vi "example_8bit_target.vi"() -> ()   [LabVIEW 2013]
uses:
  <vilib>/Platform/TimedLoop/XDataNode/wakeup.ctl
  <vilib>/Platform/TimedLoop/XDataNode/XDNodeRunTimeDep.lvlib
  <vilib>/Platform/TimedLoop/XDataNode/nitl_modes.ctl
  <vilib>/Platform/TimedLoop/XDataNode/timing_clust.ctl
  <vilib>/Platform/TimedLoop/XDataNode/XDataNode.xnode
  <vilib>/rvi/DataTransferAndStorage/Container/XNode/niFpgaContainer.xnode
  <vilib>/rvi/Memory/Memory_Emulation/niFpgaMemoryEmulationDramWriteAndRequestDataRefIn.vi
  <vilib>/eio/EIONode/EIONode.xnode
  <vilib>/rvi/eio/common/nirviEmuTemplateMethod_errors.vi
  <vilib>/rvi/FIFO/Fifo_Resource/niFpgaFifoEmulationRefIn.vi
panel:
  in  "Load":bool
  in  "Стоп":bool
  in  "Check":bool
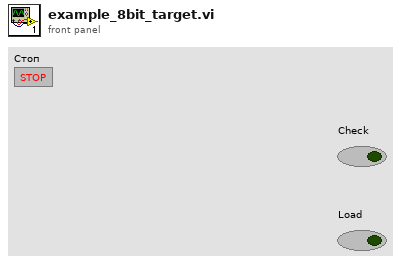
[diagram p1: front panel]
types:
  T1 = typedef "XDNodeRunTimeDep.lvlib/timing_clust.ctl" = cluster{"Expected End [f-1]":u64, "Actual End [f-1]":u64, "Finished Late? [f-1]":bool, "Expected End [i-1]":u64, "Actual End [i-1]":u64, "Finished Late? [i-1]":bool, "Expected Start [i]":u64, "Actual Start [i]":u64, "Expected Start [f]":u64, "Actual Start [f]":u64, "Source Name":string, "Structure Name":string, "Period":i64, "Deadline":i64, "Offset":i64, "Start":i64, "Priority":i32, "Timeout":i32, "Mode":T2, "Wakeup Reason":T3, "Error":errorcluster, "Source Type":string, "Secondary Source Type":string, "Global End Time":u64, "Global Start Time":u64, "Frame Duration":u64, "Iteration Duration":u64, "Assigned CPU":i32, "I/O Scan Engine Mode":u32}
  T2 = typedef "XDNodeRunTimeDep.lvlib/nitl_modes.ctl" = enum32{"No Change", "Process missed periods, maintain original phase", "Discard missed periods, maintain original phase", "Process missed periods, ignore original phase", "Discard missed periods, ignore original phase"}
  T3 = typedef "XDNodeRunTimeDep.lvlib/wakeup.ctl" = enum32{"Normal", "Aborted", "Asynchronous wakeup", "Timing source error", "Timed loop error", "Timeout"}
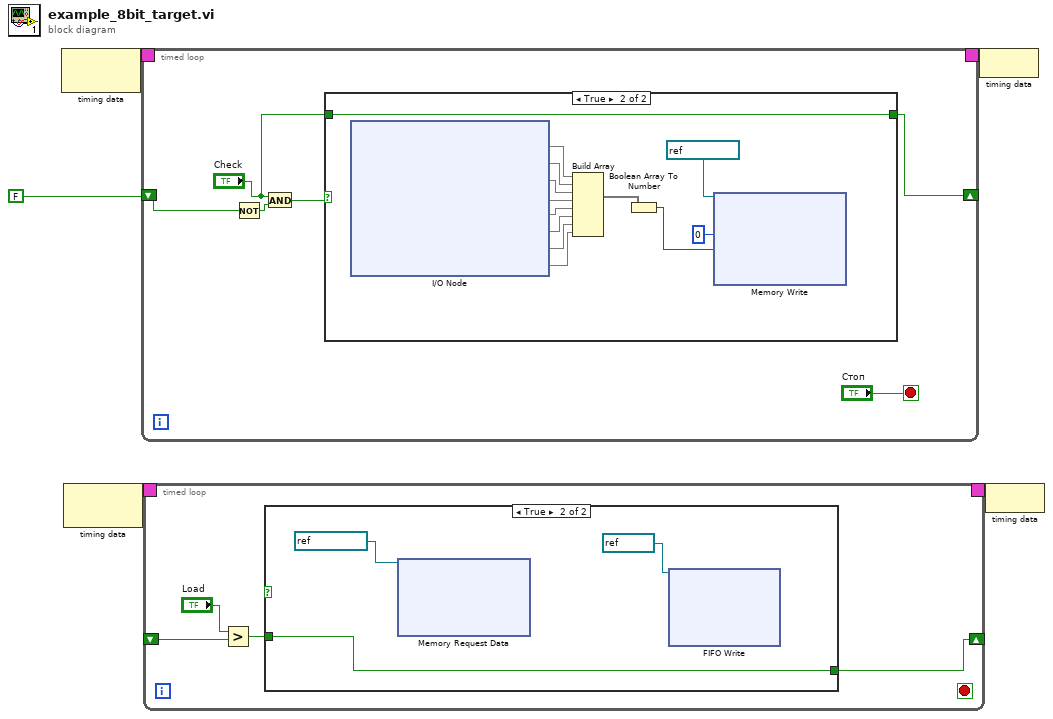
[diagram p0: block diagram]
diagram:
  n1 = node-c288() -> (w5:T1)  [unwired: 1 in]
  n2 = node-c288() -> (w3:T1)  [unwired: 1 in]
  n3 = timed-loop {
    timing: w5 -> [_]
    timing-out: [_] -> w4
    shift-right: [w7] -> _
    shift-left: FALSE -> [w8]
    stop <- "Стоп" stop-if-true
    n4 = Not(x=w8) -> (.not. x?=w9:bool)
    n5 = And(x="Check", y=w9) -> (x .and. y?=w10:bool)
    n6 = case shown="True" w10 {
      tunnel: [w12 w17] -> w7
      tunnel: "Check" -> [w12 w17]
      frame False {
      }
      frame True {
        n7 = xnode "I/O Node"() -> ("IO Module\\DDCA_DIO0_Read"=w25, "IO Module\\DDCA_DIO1_Read"=w24, "IO Module\\DDCA_DIO2_Read"=w23, "IO Module\\DDCA_DIO3_Read"=w22, "IO Module\\DDCA_DIO4_Read"=w21, "IO Module\\DDCA_DIO5_Read"=w20, "IO Module\\DDCA_DIO6_Read"=w19, "IO Module\\DDCA_DIO7_Read"=w18)  [unwired: 8 in, 8 out]
        n8 = Build Array(w25, w24, w23, w22, w21, w20, w19, w18) -> (w13:void[])
        n9 = Boolean Array To Number(Boolean array=w13) -> (number=w15:u32)
        n10 = xnode "Memory Write"("Address"=u32 0, "Data"=w15, "Memory In"=refnum<k21> "Memory") -> ()  [unwired: 1 in, 2 out]
      }
    }
  }
  n11 = timed-loop {
    timing: w3 -> [_]
    timing-out: [_] -> w2
    shift-right: [w30] -> _
    shift-left: _ -> [w28]
    stop <- _ stop-if-true
    n12 = Greater?(x="Load", y=w28) -> (0:w29:bool)
    n13 = case shown="True" {
      selector: _ -> [_ _]
      tunnel: [_ w32] -> w30
      tunnel: w29 -> [_ w32]
      frame False {
      }
      frame True {
        n14 = xnode "Memory Request Data"("Memory In"=refnum<k21> "Memory") -> ()  [unwired: 2 in, 2 out]
        n15 = xnode "FIFO Write"("FIFO In"=refnum<k21> "FIFO") -> ()  [unwired: 2 in, 2 out]
      }
    }
  }
  n16 = node-c288(w4) -> ()
  n17 = node-c288(w2) -> ()
